vi "Process Digital Pattern.vi"(0 "EPT Pattern":T2, 5 "Rotations":u16) -> (2 "Base Repeats":i32, 3 "Base Teeth":dbl[](array[numeric]), 4 "Base":T1, 6 "Reduced":T1, 8 "Final":T1, 13 "Final":bool, 14 "Reduced":bool)   [LabVIEW 2013, in "Engine Simulation Toolkit System Explorer.lvlib"]
uses:
  Engine Simulation Toolkit System Explorer.lvlib
  Digital Pattern.ctl
  Digital Pattern Base.ctl
  Digital Pattern Remove Edge.ctl
  Digital Pattern Add Pulse.ctl
  Digital Pattern Expanded.ctl
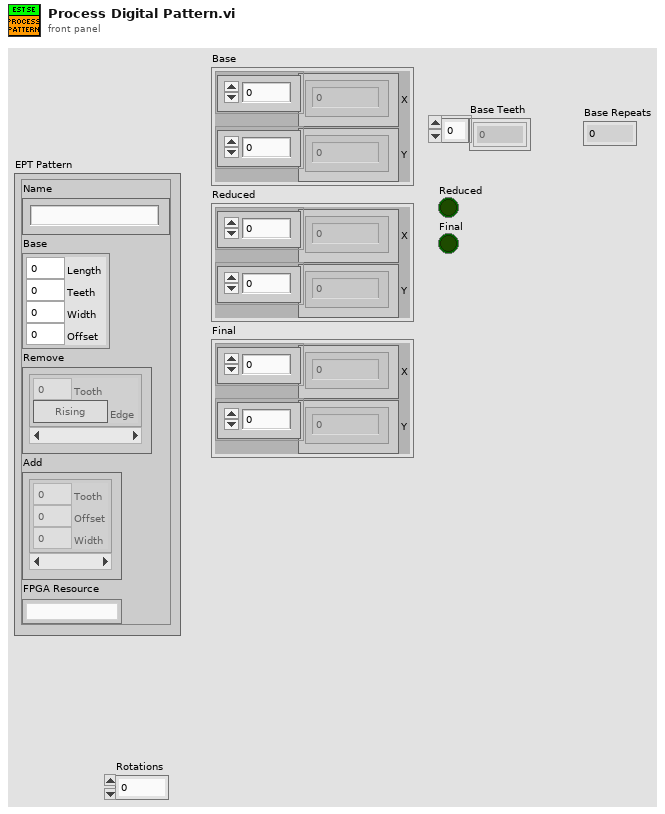
[diagram p1: front panel]
types:
  T1 = typedef "Engine Simulation Toolkit System Explorer.lvlib/Digital Pattern Expanded.ctl" = cluster{"X":dbl[], "Y":dbl[]}
  T2 = typedef "Engine Simulation Toolkit System Explorer.lvlib/Digital Pattern.ctl" = cluster{"Name":string, "Base":T3, "Remove":T4[], "Add":T5[], "FPGA Resource":string}
  T3 = typedef "Engine Simulation Toolkit System Explorer.lvlib/Digital Pattern Base.ctl" = cluster{"Length":dbl, "Teeth":u16, "Width":dbl, "Offset":dbl}
  T4 = typedef "Engine Simulation Toolkit System Explorer.lvlib/Digital Pattern Remove Edge.ctl" = cluster{"Tooth":u16, "Edge":bool}
  T5 = typedef "Engine Simulation Toolkit System Explorer.lvlib/Digital Pattern Add Pulse.ctl" = cluster{"Tooth":u16, "Offset":dbl, "Width":dbl}
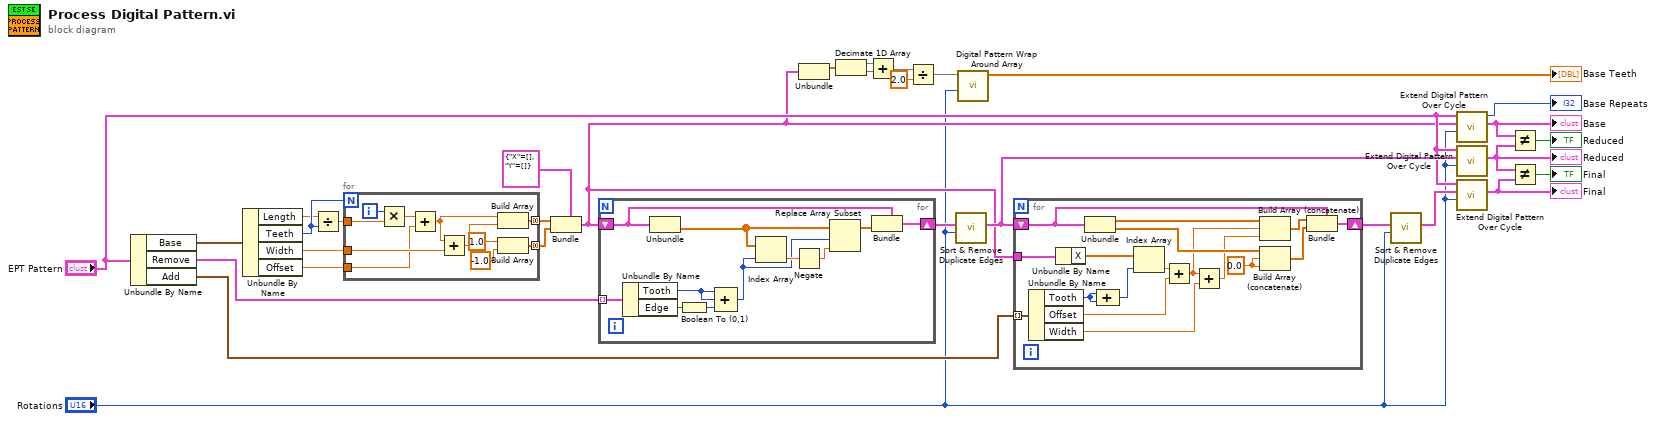
[diagram p0: block diagram]
diagram:
  n1 = Unbundle By Name("EPT Pattern") -> ("Base"=w24:T3, "Remove"=w27:T4[], "Add"=w30:T5[])
  n2 = Unbundle By Name(w24) -> ("Length"=w2:dbl, "Teeth"=w25:u16, "Width"=w26:dbl, "Offset"=w6:dbl)
  n3 = Divide(x=w2, y=w25) -> (x/y=w23:dbl)
  n4 = for {
    N: w25 -> [_]
    tunnel: w23 -> [w40]
    tunnel: w26 -> [w41]
    tunnel: [w36] -> w21 mode=concatenating
    tunnel: [w35] -> w22 mode=concatenating
    tunnel: w6 -> [w32]
    i -> [w42]
    n5 = Multiply(x=w42, y=w40) -> (x*y=w34:dbl)
    n6 = Add(x=w34, y=w32) -> (x+y=w33:dbl)
    n7 = Add(x=w33, y=w41) -> (x+y=w39:dbl)
    n8 = Build Array(w33, w39) -> (w35:dbl[])
    n9 = Build Array(1.0, -1.0) -> (w36:dbl[])
  }
  n10 = Bundle(cluster=T1 {"X"=[], "Y"=[]} ("Base Pattern"), "X"=w22, "Y"=w21) -> (w7:T1)
  n11 = for {
    shift-right: [w53] -> w29
    shift-left: w7 -> [w52]
    tunnel: w27 -> [w47] mode=indexing
    n12 = Unbundle By Name(w47) -> ("Tooth"=w44:u16, "Edge"=w46:bool)
    n13 = Unbundle(w52) -> ("Y"=w50:dbl[])  [unwired: 1 out]
    n14 = Boolean To (0,1)(Boolean=w46) -> (0, 1=w45:i16)
    n15 = Compound Arithmetic op=ADD(w44, w44, w45) -> (w43:u16)
    n16 = Index Array(array=w50, index=w43) -> (element=w48:dbl)
    n17 = Negate(x=w48) -> (-x=w49:dbl)
    n18 = Replace Array Subset(array=w50, new element=w49, index=w43) -> (w51:dbl[])
    n19 = Bundle(cluster=w52, "Y"=w51) -> (w53:T1)  [unwired: 1 in]
  }
  n20 = Unbundle(w7) -> ("X"=w14:dbl[])  [unwired: 1 out]
  n21 = Decimate 1D Array(w14) -> (w13:dbl[], w12:dbl[])
  n22 = Add(x=w13, y=w12) -> (x+y=w11:dbl[])
  n23 = Divide(x=w11, y=2.0) -> (x/y=w9:dbl[])
  n24 = call "Sort & Remove Duplicate Edges.vi"("Rotations"="Rotations", "Pattern"=w29) -> ("Pattern"=w18:T1)  [unwired: 9 in]
  n25 = call "Digital Pattern Wrap Around Array.vi"("Rotations"="Rotations", "x"=w9) -> ("x"=→"Base Teeth":dbl[])  [unwired: 9 in]
  n26 = for {
    shift-right: [w70] -> w31
    shift-left: w18 -> [w69]
    tunnel: w30 -> [w68] mode=indexing
    tunnel: w7 -> [w63]
    w56 = 0.0
    n27 = Unbundle By Name(w68) -> ("Tooth"=w55:u16, "Offset"=w60:dbl, "Width"=w58:dbl)
    n28 = Unbundle By Name(w63) -> ("X"=w62:dbl[])
    n29 = Unbundle(w69) -> ("X"=w67:dbl[], "Y"=w65:dbl[])
    n30 = Compound Arithmetic op=ADD(w55, w55) -> (w54:u16)
    n31 = Index Array(array=w62, index=w54) -> (element=w61:dbl)
    n32 = Add(x=w61, y=w60) -> (x+y=w59:dbl)
    n33 = Add(x=w59, y=w58) -> (x+y=w57:dbl)
    n34 = Build Array (concatenate)(w67, w59, w57) -> (w66:dbl[])
    n35 = Build Array (concatenate)(w65, w56, w56) -> (w64:dbl[])
    n36 = Bundle(cluster=w69, "X"=w66, "Y"=w64) -> (w70:T1)
  }
  n37 = call "Sort & Remove Duplicate Edges.vi"("Rotations"="Rotations", "Pattern"=w31) -> ("Pattern"=w4:T1)  [unwired: 9 in]
  n38 = call "Extend Digital Pattern Over Cycle.vi"("Rotations"="Rotations", "Pattern"=w7, "EPT Pattern"="EPT Pattern") -> ("Pattern"=w17:T1, "Base Repeats"=→"Base Repeats":i32)  [unwired: 7 in]
  "Base" <- w17
  n39 = call "Extend Digital Pattern Over Cycle.vi"("Rotations"="Rotations", "Pattern"=w18, "EPT Pattern"="EPT Pattern") -> ("Pattern"=w16:T1)  [unwired: 7 in, 1 out]
  "Reduced" <- w16
  n40 = call "Extend Digital Pattern Over Cycle.vi"("Rotations"="Rotations", "Pattern"=w4, "EPT Pattern"="EPT Pattern") -> ("Pattern"=w5:T1)  [unwired: 7 in, 1 out]
  "Final" <- w5
  n41 = Not Equal?(x=w17, y=w16) -> (x != y?=→"Reduced":bool)
  n42 = Not Equal?(x=w16, y=w5) -> (x != y?=→"Final":bool)
